vi "LogError.vi"(8 "error in (no error)":errorcluster, 10 "ErrorToLog":errorcluster, 11 "object in":refnum<class "EventLogger_Actor.lvclass">) -> (0 "error out":errorcluster, 3 "object out":refnum<class "EventLogger_Actor.lvclass">)   [LabVIEW 2014, in "EventLogger_Actor.lvlib" / "EventLogger_Actor.lvclass"]
uses:
  EventLogger_Actor.lvclass
  <vilib>/Utility/error.llb/DialogType.ctl
  EventLogger_Actor.lvclass/EventLogger_Actor.ctl
  <userlib>/_OpenG.lib/string/string.llb/Trim Whitespace (String)__ogtk.vi
panel:
  # "BSD 2-Clause License\n\nCopyright (c) 2018, Ajay www.digiajay.com\nAll rights reserved.\n\nRedistribution and use in source and binary forms, with or without\nmodification, are permitted provided that the following conditions are met:\n\n* Redistributions of source code must retain the above copyright notice, this\n  list of conditions and the following disclaimer.\n\n* Redistributions in binary form must reproduce the above copyright notice,\n  this list of conditions and the following disclaimer in the documentation\n  and/or other materials provided with the distribution.\n\nTHIS SOFTWARE IS PROVIDED BY THE COPYRIGHT HOLDERS AND CONTRIBUTORS \"AS IS\"\nAND ANY EXPRESS OR IMPLIED WARRANTIES, INCLUDING, BUT NOT LIMITED TO, THE\nIMPLIED WARRANTIES OF MERCHANTABILITY AND FITNESS FOR A PARTICULAR PURPOSE ARE\nDISCLAIMED. IN NO EVENT SHALL THE COPYRIGHT HOLDER OR CONTRIBUTORS BE LIABLE\nFOR ANY DIRECT, INDIRECT, INCIDENTAL, SPECIAL, EXEMPLARY, OR CONSEQUENTIAL\nDAMAGES (INCLUDING, BUT NOT LIMITED TO, PROCUREMENT OF SUBSTITUTE GOODS OR\nSERVICES; LOSS OF USE, DATA, OR PROFITS; OR BUSINESS INTERRUPTION) HOWEVER\nCAUSED AND ON ANY THEORY OF LIABILITY, WHETHER IN CONTRACT, STRICT LIABILITY,\nOR TORT (INCLUDING NEGLIGENCE OR OTHERWISE) ARISING IN ANY WAY OUT OF THE USE\nOF THIS SOFTWARE, EVEN IF ADVISED OF THE POSSIBILITY OF SUCH DAMAGE."
  # "Connector Pane"
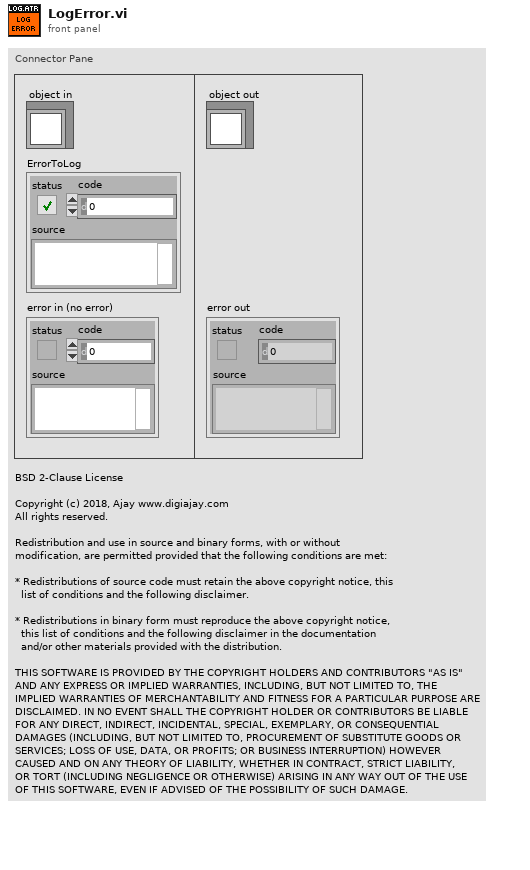
[diagram p1: front panel]
types:
  T1 = typedef "DialogType.ctl" = u16
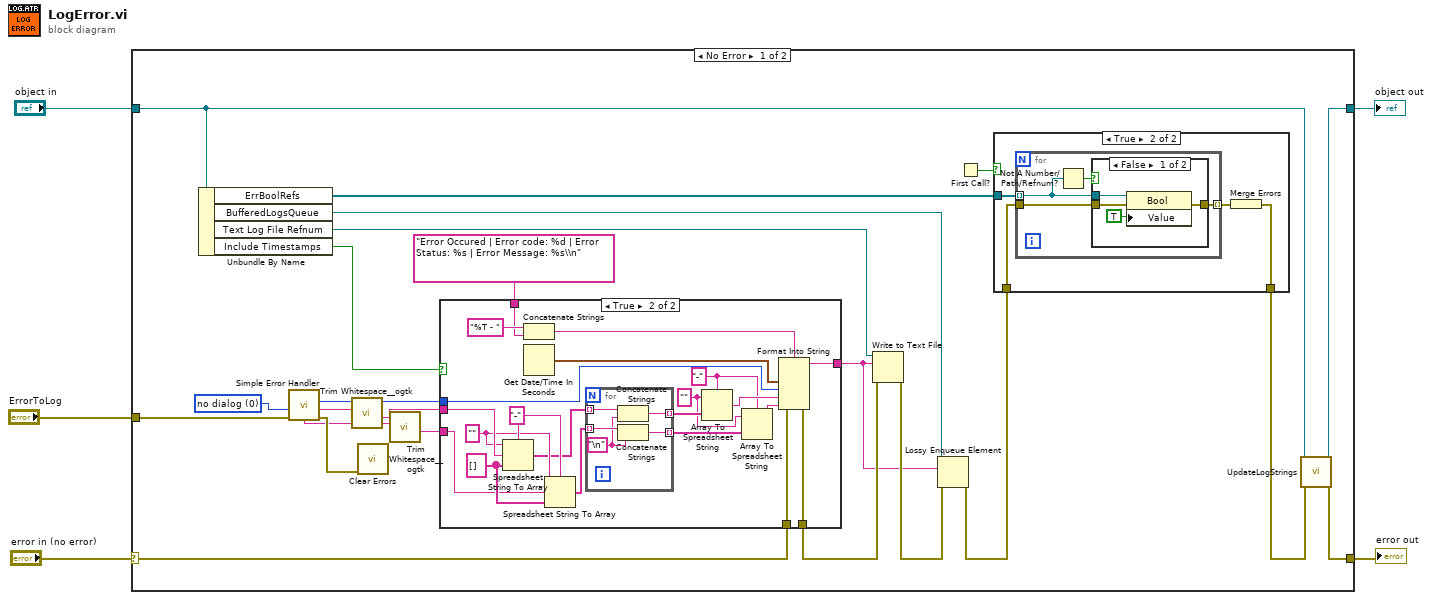
[diagram p0: block diagram]
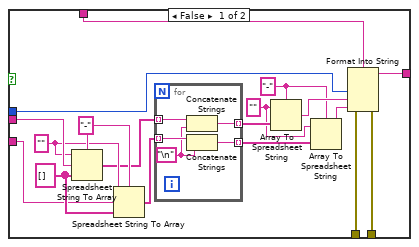
[diagram p4: hidden frame]
diagram:
  n1 = case shown="No Error" "error in (no error)" {
    selector: "error in (no error)" -> [w27 w93]
    tunnel: [w8 w93] -> w4
    tunnel: [w7 w92] -> w2
    tunnel: "object in" -> [w6 w92]
    tunnel: "ErrorToLog" -> [w26 _]
    frame No Error {
      w25 = T1 0 items=["no dialog", "OK message", "continue or stop message", "OK message + warnings", "continue/stop + warnings"] ("type of dialog (OK msg:1)")
      n2 = Unbundle By Name(w6) -> ("ErrBoolRefs"=w15:refnum<vi>[], "BufferedLogsQueue"=w10:refnum<queue>, "Text Log File Refnum"=w17:refnum<file>, "Include Timestamps"=w18:bool)
      n3 = call <vilib>:"Simple Error Handler.vi"("type of dialog (OK msg:1)"=w25, "error in (no error)"=w26) -> ("code out"=w24:i32, "source out"=w23:string, "error out"=w22:errorcluster, "message"=w20:string)  [unwired: 3 in, 1 out]
      n4 = call-poly <userlib>:"Trim Whitespace__ogtk.vi"("String in"=w23) -> ("String out"=w21:string)  [unwired: 6 in]
      n5 = call <vilib>:"Clear Errors.vi"("error in (no error)"=w22) -> ()  [unwired: 5 in, 2 out]
      n6 = call-poly <userlib>:"Trim Whitespace__ogtk.vi"("String in"=w20) -> ("String out"=w19:string)  [unwired: 6 in]
      n7 = case shown="True" w18 {
        tunnel: "Error Occured | Error code: %d | Error Status: %s | Error Message: %s\\n" ("format string") -> [w43 w69]
        tunnel: w27 -> [w46 w72]
        tunnel: [w45 w71] -> w16
        tunnel: [w47 w73] -> w9
        tunnel: w24 -> [w44 w68]
        tunnel: w21 -> [w59 w85]
        tunnel: w19 -> [w58 w84]
        frame False {
          w48 = ""
          w49 = "-" ("delimiter (Tab)")
          w56 = ""
          w60 = string[] [] ("delimiter (Tab)")
          w57 = "-" ("delimiter (Tab)")
          n8 = Spreadsheet String To Array(delimiter (Tab)=w57, format string=w56, spreadsheet string=w59, array type (2D Dbl)=w60) -> (array=w55:string[])
          n9 = Spreadsheet String To Array(delimiter (Tab)=w57, format string=w56, spreadsheet string=w58, array type (2D Dbl)=w60) -> (array=w54:string[])
          n10 = for {
            tunnel: w55 -> [w65] mode=indexing
            tunnel: w54 -> [w64] mode=indexing
            tunnel: [w62] -> w53 mode=indexing
            tunnel: [w61] -> w52 mode=indexing
            w63 = "\n"
            n11 = Concatenate Strings(w65, w63) -> (w62:string)
            n12 = Concatenate Strings(w64, w63) -> (w61:string)
          }
          n13 = Array To Spreadsheet String(delimiter (Tab)=w49, array=w53, 3:w48) -> (spreadsheet string=w51:string)
          n14 = Array To Spreadsheet String(delimiter (Tab)=w49, array=w52, 3:w48) -> (spreadsheet string=w50:string)
          n15 = Format Into String(format string=w43, error in=w46, w44, w51, w50) -> (resulting string=w47:string, error out=w45:errorcluster)  [unwired: 1 in]
        }
        frame True {
          w74 = ""
          w75 = "-" ("delimiter (Tab)")
          w82 = ""
          w86 = string[] [] ("delimiter (Tab)")
          w83 = "-" ("delimiter (Tab)")
          n16 = Spreadsheet String To Array(delimiter (Tab)=w83, format string=w82, spreadsheet string=w85, array type (2D Dbl)=w86) -> (array=w81:string[])
          n17 = Concatenate Strings("%T - " ("string"), w69) -> (w66:string)
          n18 = Get Date/Time In Seconds() -> (seconds since 1Jan1904=w67:timestamp)
          n19 = Spreadsheet String To Array(delimiter (Tab)=w83, format string=w82, spreadsheet string=w84, array type (2D Dbl)=w86) -> (array=w80:string[])
          n20 = for {
            tunnel: w81 -> [w91] mode=indexing
            tunnel: w80 -> [w90] mode=indexing
            tunnel: [w88] -> w79 mode=indexing
            tunnel: [w87] -> w78 mode=indexing
            w89 = "\n"
            n21 = Concatenate Strings(w91, w89) -> (w88:string)
            n22 = Concatenate Strings(w90, w89) -> (w87:string)
          }
          n23 = Array To Spreadsheet String(delimiter (Tab)=w75, array=w79, 3:w74) -> (spreadsheet string=w77:string)
          n24 = Array To Spreadsheet String(delimiter (Tab)=w75, array=w78, 3:w74) -> (spreadsheet string=w76:string)
          n25 = Format Into String(format string=w66, error in=w72, w67, w68, w77, w76) -> (resulting string=w73:string, error out=w71:errorcluster)  [unwired: 1 in]
        }
      }
      n26 = Write to Text File(file (use dialog)=w17, text=w9, error in=w16) -> (error out=w14:errorcluster)  [unwired: 1 in, 2 out]
      n27 = Lossy Enqueue Element(queue=w10, element=w9, error in (no error)=w14) -> (error out=w11:errorcluster)  [unwired: 3 out]
      n28 = First Call?() -> (First Call?: T/F=w12:bool)
      n29 = case shown="True" w12 {
        tunnel: w15 -> [_ w33]
        tunnel: w11 -> [w29 w32]
        tunnel: [w29 w30] -> w13
        frame False {
        }
        frame True {
          n30 = for {
            tunnel: w33 -> [w36] mode=indexing
            tunnel: w32 -> [w35]
            tunnel: [w37] -> w31 mode=indexing
            n31 = Not A Number/Path/Refnum?(number/path/refnum=w36) -> (NaN/Path/Refnum?=w34:bool)
            n32 = case shown="False" w34 {
              tunnel: [w40 w42] -> w37
              tunnel: w36 -> [w39 _]
              tunnel: w35 -> [w38 w42]
              frame False {
                n33 = property class="Bool"(reference=w39, error in=w38, "Value"=TRUE) -> (error out=w40:errorcluster)  [unwired: 1 out]
              }
              frame True {
              }
            }
          }
          n34 = Merge Errors(w31) -> (w30:errorcluster)
        }
      }
      n35 = call "UpdateLogStrings.vi"("error in (no error)"=w13, "object in"=w6) -> ("error out"=w8:errorcluster, "object out"=w7:refnum<class "EventLogger_Actor.lvclass">)  [unwired: 8 in]
    }
    frame Error {
    }
  }
  "error out" <- w4
  "object out" <- w2
